vi "PeriodicFilter-Auto Set Filter.vi"(11 "Data In":T1 {"LastCheckT" format="%<%.3X>T"}) -> (3 "Data Out":T1 {"LastCheckT" format="%<%.3X>T"})   [LabVIEW 2017, in "Communicable State Machine.lvlib"]
uses:
  Communicable State Machine.lvlib
  Periodic String Filter Data.ctl
  Periodic String Filter Info.ctl
  _Support/Typedef/_CSM_GlobalLog_MSG_TYPE.ctl
  _Support/GlobalEvent/GEvt-Set Source Filter Rules - v1.2.vi
  _Shared/CSM Shared.lvlib
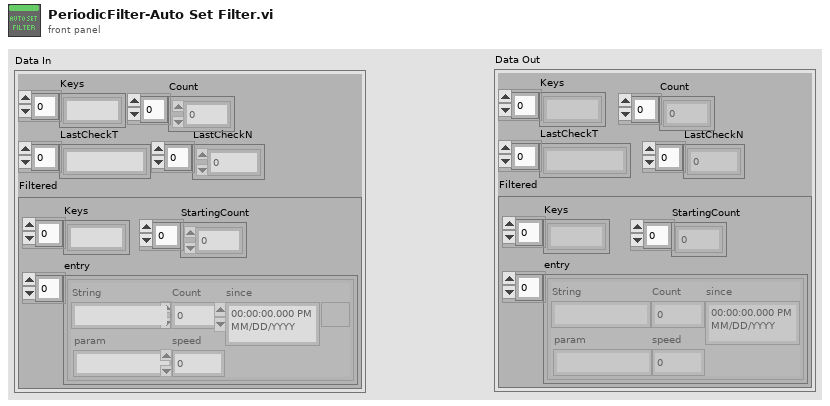
[diagram p1: front panel]
types:
  T1 = typedef "Communicable State Machine.lvlib/Periodic String Filter Data.ctl" = cluster{"Keys":string[], "Count":i64[], "LastCheckT":timestamp[], "LastCheckN":i64[], "Filtered":cluster{"Keys":string[], "StartingCount":i64[], "entry":T2[]}}
  T2 = typedef "Communicable State Machine.lvlib/Periodic String Filter Info.ctl" = cluster{"String":string, "Count":i64, "since":timestamp, "param":string, "speed":dbl}
  T3 = typedef "Communicable State Machine.lvlib/_CSM_GlobalLog Filter Rules - v1.2.ctl" = cluster{"Global":cluster{"CSM":string[], "LogType":T4[], "State":string[], "StateType":T5[], "Broadcast":string[]}, "CSM":cluster{"LogType":cluster{"CSM":string, "LogType":T4}[], "State":cluster{"CSM":string, "State":string}[], "StateType":cluster{"CSM":string, "LogType":T5}[], "Broadcast":cluster{"CSM":string, "Broadcast":string}[]}, "PeriodicMessageFilter":cluster{"Enable":bool, "Threshold(#/s)":dbl, "CheckPeriod(s)":dbl}}
  T4 = typedef "Communicable State Machine.lvlib/_CSM_GlobalLog_MSG_TYPE.ctl" = enum16{"User Log", "State Change", "Status", "Interrupt", "Register", "Unregister", "Error Log", "Module Created", "Module Destroyed", "Async Message", "No-Rep Async Message", "Sync Message", "AsyncMsg Complete", "SyncMsg Complete"}
  T5 = typedef "Communicable State Machine.lvlib/_CSM_GlobalLog_STATE_TYPE.ctl" = enum16{"State - Internal State", "State - External Message", "State - Response", "State - Complete"}
  T6 = cluster{"CSM":string[], "LogType":T4[], "State":string[], "StateType":T5[], "Broadcast":string[]}
  T7 = cluster{"LogType":cluster{"CSM":string, "LogType":T4}[], "State":cluster{"CSM":string, "State":string}[], "StateType":cluster{"CSM":string, "LogType":T5}[], "Broadcast":cluster{"CSM":string, "Broadcast":string}[]}
  T8 = cluster{"trimed text":string, "trimed text":string}
  T9 = cluster{"Global":cluster{"CSM":string[], "LogType":T4[], "State":string[], "StateType":T5[], "Broadcast":string[]}, "CSM":cluster{"LogType":cluster{"CSM":string, "LogType":T4}[], "State":cluster{"CSM":string, "State":string}[], "StateType":cluster{"CSM":string, "LogType":T5}[], "Broadcast":cluster{"CSM":string, "Broadcast":string}[]}}
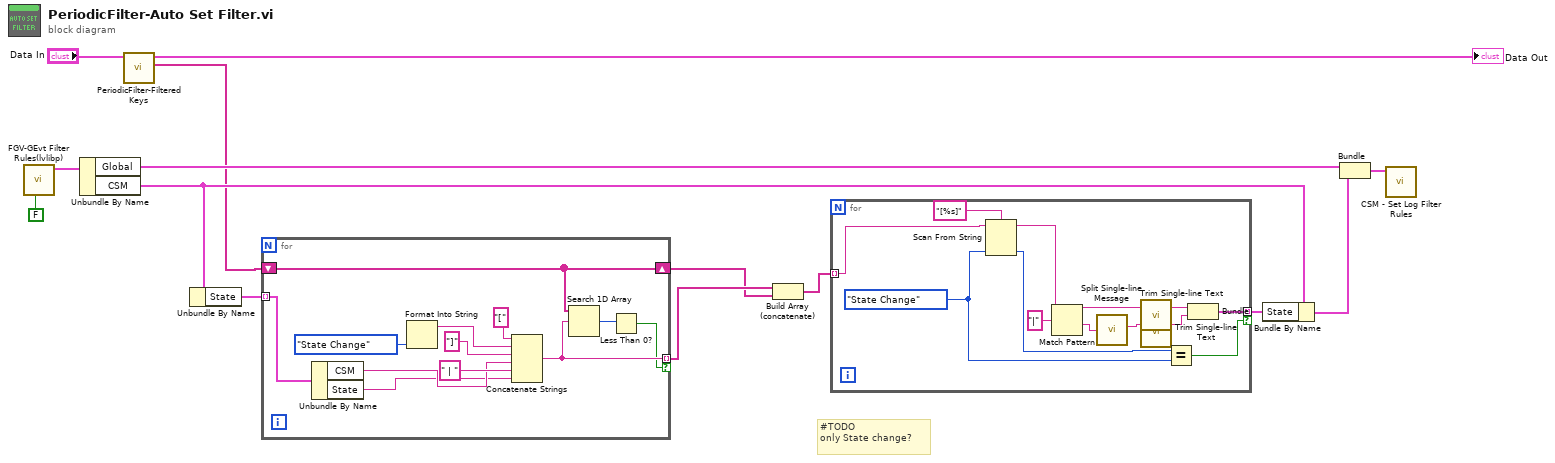
[diagram p0: block diagram]
diagram:
  # "#TODO\nonly State change?"
  n1 = call "FGV-GEvt Filter Rules(lvlibp).vi"("Set? (T)/Get(F)"=FALSE ("Set(T)/Get(F)")) -> ("Rules-v1.2 out"=w1:T3)  [unwired: 9 in, 1 out]
  n2 = Unbundle By Name(w1) -> ("Global"=w12:T6, "CSM"=w6:T7)
  n3 = call "PeriodicFilter-Filtered Keys.vi"("Data In"="Data In") -> ("Filtered Keys"=w4:string[], "Data Out"=→"Data Out":T1)  [unwired: 9 in]
  n4 = Unbundle By Name(w6) -> ("State"=w5:cluster{"CSM":string, "State":string}[])
  n5 = for {
    tunnel: w5 -> [w22] mode=indexing
    tunnel: [w17] -> w3 mode=indexing if=w15
    shift-right: [w18] -> w2
    shift-left: w4 -> [w18]
    n6 = Unbundle By Name(w22) -> ("CSM"=w21:string, "State"=w20:string)
    n7 = Format Into String(_CSM_GlobalLog_MSG_TYPE."State Change" ("input 1")) -> (resulting string=w23:string)  [unwired: 3 in, 1 out]
    n8 = Concatenate Strings("[" ("string"), w23, "]" ("string"), w21, " | " ("string"), w20) -> (w17:string)
    n9 = Search 1D Array(1D array=w18, element=w17) -> (index of element=w16:i32)  [unwired: 1 in]
    n10 = Less Than 0?(x=w16) -> (x < 0?=w15:bool)
  }
  n11 = Build Array (concatenate)(w3, w2) -> (w7:string[])
  n12 = for {
    tunnel: [w37] -> w13 mode=indexing if=w36
    tunnel: w7 -> [w27] mode=indexing
    w34 = _CSM_GlobalLog_MSG_TYPE."State Change" ("LogType")
    n13 = Scan From String(format string="[%s]", input string=w27, default 1=w34) -> (remaining string=w33:string, output 1=w28:T4)  [unwired: 2 in, 2 out]
    n14 = Match Pattern(string=w33, regular expression="|") -> (before substring=w31:string, after substring=w30:string)  [unwired: 1 in, 2 out]
    n15 = call "Split Single-line Message.vi"("single-line text"=w30) -> ("state"=w29:string)  [unwired: 6 in, 3 out]
    n16 = call "Trim Single-line Text.vi"("single-line text"=w31) -> ("trimed text"=w39:string)  [unwired: 2 in]
    n17 = call "Trim Single-line Text.vi"("single-line text"=w29) -> ("trimed text"=w38:string)  [unwired: 2 in]
    n18 = Equal?(x=w28, y=w34) -> (x = y?=w36:bool)
    n19 = Bundle("trimed text"=w39, "trimed text"=w38) -> (w37:T8)  [unwired: 1 in]
  }
  n20 = Bundle By Name(cluster=w6, "State"=w13) -> (w11:T7)
  n21 = Bundle("Global"=w12, "CSM"=w11) -> (w10:T9)  [unwired: 1 in]
  n22 = call-poly "CSM - Set Log Filter Rules.vi"("Rules-v1.2"=w10) -> ()  [unwired: 10 in, 1 out]
